vi "Post_request.vi"   [LabVIEW 2016]
uses:
  Headers/Headers.ctl
types:
  T1 = typedef "Headers.ctl" = cluster{"Name":string, "Value":string}[]
  T2 = typedef "URL_Data.ctl" = cluster{"Root":string, "Endpoint":string, "Request_URL":string}
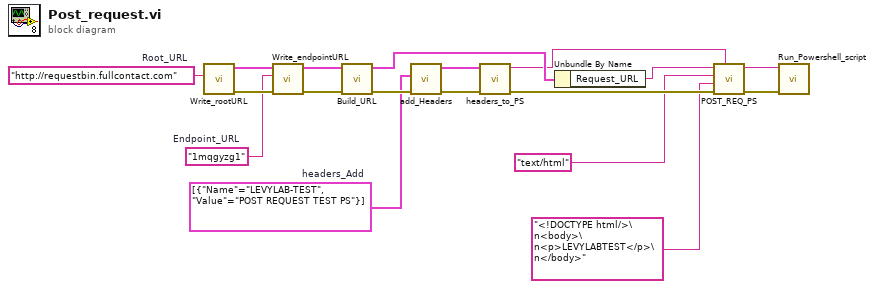
[diagram p0: block diagram]
diagram:
  w6 = T1 [{"Name"="LEVYLAB-TEST", "Value"="POST REQUEST TEST PS"}]  # headers_Add
  w8 = "1mqgyzg1"  # Endpoint_URL
  w9 = "http://requestbin.fullcontact.com"  # Root_URL
  n1 = call "Write_rootURL.vi"("Root_URL"=w9) -> ("error out"=w10:errorcluster, "URL OUT"=w18:T2)  [unwired: 9 in]
  n2 = call "Write_endpointURL.vi"("error in"=w10, "Endpoint_URL"=w8, "URL IN"=w18) -> ("error out"=w11:errorcluster, "URL OUT"=w17:T2)  [unwired: 7 in]
  n3 = call "Build_URL.vi"("error in"=w11, "URL IN"=w17) -> ("error out"=w12:errorcluster, "URL OUT"=w16:T2)  [unwired: 8 in]
  n4 = call "add_Headers.vi"("error in"=w12, "headers_Add"=w6) -> ("error out"=w13:errorcluster, "Headers Out"=w7:T1)  [unwired: 8 in]
  n5 = call "headers_to_PS.vi"("error in"=w13, "Headers In"=w7) -> ("error out"=w14:errorcluster, "Headers_PS_Dict"=w3:string)  [unwired: 8 in]
  n6 = Unbundle By Name(w16) -> ("Request_URL"=w15:string)
  n7 = call "POST_REQ_PS.vi"("Headers"=w3, "error in"=w14, "Body"="<!DOCTYPE html/>\n<body>\n<p>LEVYLABTEST</p>\n</body>", "ContentType"="text/html", "URL"=w15) -> ("error out"=w4:errorcluster, "POST Request"=w5:string)  [unwired: 5 in]
  n8 = call "Run_Powershell_script.vi"("error in"=w4, "Powershell Script"=w5) -> ()  [unwired: 7 in, 3 out]
